vi "sgp4.vi"(5 "UTC":dbl, 6 "TLE":string) -> (2 "r":T1)   [LabVIEW 2015]
uses:
  <vilib>/Analysis/Matrix/Datatypes/RealMatrix.ctl
  <vilib>/Analysis/Matrix/NI_Matrix.lvlib
panel:
  out "Line 1":string
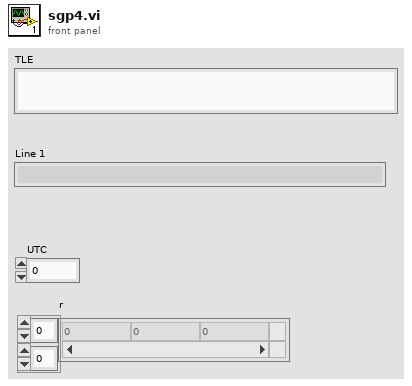
[diagram p1: front panel]
types:
  T1 = typedef "NI_Matrix.lvlib/RealMatrix.ctl" = dbl[][]
  T2 = cluster{"sinmao":sgl, "t":sgl, "t2cof":sgl, "t3cof":sgl, "t4cof":sgl, "t5cof":sgl, "x1mth2":sgl, "x7thm1":sgl, "mdot":sgl, "nodedot":sgl, "xlcof":sgl, "xmcof":sgl, "nodecf":sgl, "irez":sgl, "d2201":sgl, "d2211":sgl, "d3210":sgl, "d3222":sgl, "d4410":sgl, "d4422":sgl, "d5220":sgl, "d5232":sgl, "d5421":sgl, "d5433":sgl, "dedt":sgl, "del1":sgl, "del2":sgl, "del3":sgl, "didt":sgl, "dmdt":sgl, "dnodt":sgl, "domdt":sgl, "e3":sgl, "ee2":sgl, "peo":sgl, "pgho":sgl, "pho":sgl, "pinco":sgl, "plo":sgl, "se2":sgl, "se3":sgl, "sgh2":sgl, "sgh3":sgl, "sgh4":sgl, "sh2":sgl, "sh3":sgl, "si2":sgl, "si3":sgl, "sl2":sgl, "sl3":sgl, "sl4":sgl, "gsto":sgl, "xfact":sgl, "xgh2":sgl, "xgh3":sgl, "xgh4":sgl, "xh2":sgl, "xh3":sgl, "xi2":sgl, "xi3":sgl, "xl2":sgl, "xl3":sgl, "xl4":sgl, "xlamo":sgl, "zmol":sgl, "zmos":sgl, "atime":sgl, "xli":sgl, "xni":sgl, "init":string[], "error":sgl, "satnum":cdb, "epochyr":cdb, "epochdays":cdb, "ndot":cdb, "nddot":cdb, "bstar":cdb, "inclo":cdb, "nodeo":cdb, "ecco":cdb, "argpo":cdb, "mo":cdb, "a":cdb, "alta":cdb, "altp":cdb, "isimp":sgl, "method":string[], "aycof":sgl, "con41":sgl, "cc1":sgl, "cc4":sgl, "cc5":sgl, "d2":sgl, "d3":sgl, "d4":sgl, "delmo":sgl, "eta":sgl, "argpdot":sgl, "omgcof":sgl, "no":cdb, "jdsatepoch":dbl}
  T3 = cluster{"sinmao":cdb, "t":dbl, "t2cof":cdb, "t3cof":cdb, "t4cof":cdb, "t5cof":cdb, "x1mth2":cdb, "x7thm1":cdb, "mdot":cdb, "nodedot":cdb, "xlcof":cdb, "xmcof":cdb, "nodecf":cdb, "irez":sgl, "d2201":dbl, "d2211":dbl, "d3210":dbl, "d3222":dbl, "d4410":dbl, "d4422":dbl, "d5220":dbl, "d5232":dbl, "d5421":dbl, "d5433":dbl, "dedt":dbl, "del1":dbl, "del2":dbl, "del3":dbl, "didt":dbl, "dmdt":dbl, "dnodt":dbl, "domdt":dbl, "e3":cdb, "ee2":cdb, "peo":dbl, "pgho":dbl, "pho":dbl, "pinco":dbl, "plo":dbl, "se2":cdb, "se3":cdb, "sgh2":cdb, "sgh3":cdb, "sgh4":cdb, "sh2":cdb, "sh3":cdb, "si2":cdb, "si3":cdb, "sl2":cdb, "sl3":cdb, "sl4":cdb, "gsto":dbl, "xfact":dbl, "xgh2":cdb, "xgh3":cdb, "xgh4":cdb, "xh2":cdb, "xh3":cdb, "xi2":cdb, "xi3":cdb, "xl2":cdb, "xl3":cdb, "xl4":cdb, "xlamo":dbl, "zmol":dbl, "zmos":dbl, "atime":dbl, "xli":dbl, "xni":dbl, "init":string[], "error":sgl, "satnum":sgl, "epochyr":sgl, "epochdays":dbl, "ndot":dbl, "nddot":dbl, "bstar":dbl, "inclo":cdb, "nodeo":cdb, "ecco":cdb, "argpo":cdb, "mo":cdb, "a":cdb, "alta":cdb, "altp":cdb, "isimp":sgl, "method":string[], "aycof":cdb, "con41":cdb, "cc1":cdb, "cc4":cdb, "cc5":cdb, "d2":cdb, "d3":cdb, "d4":cdb, "delmo":cdb, "eta":cdb, "argpdot":cdb, "omgcof":cdb, "no":cdb, "jdsatepoch":dbl}
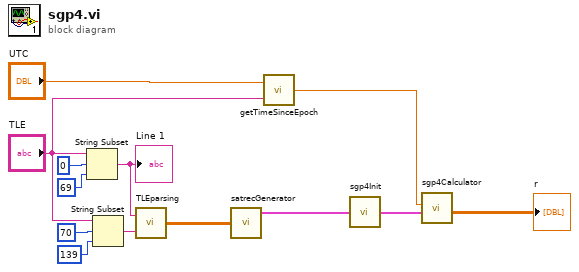
[diagram p0: block diagram]
diagram:
  n1 = String Subset(string="TLE", offset (0)=0, length (rest)=69) -> (substring=w8:string)
  "Line 1" <- w8
  n2 = String Subset(string="TLE", offset (0)=70, length (rest)=139) -> (substring=w7:string)
  n3 = call "TLEparsing.vi"("String 2"=w7, "String"=w8) -> ("parametres_TLE"=w13:cdb[][])
  n4 = call "satrecGenerator.vi"("parametres_TLE"=w13) -> ("satrec"=w6:T2)  [unwired: 2 in, 2 out]
  n5 = call "getTimeSinceEpoch.vi"("TLE"="TLE", "UTC"="UTC") -> ("number of minutes since\nthe epoch (t-t0) (min)"=w1:dbl)
  n6 = call "sgp4Init.vi"("satrec"=w6) -> ("satrec 2"=w5:T3)
  n7 = call "sgp4Calculator.vi"("output cluster"=w5, "tsince"=w1) -> ("r"=→"r":cdb[][])  [unwired: 7 in, 2 out]
